vi "Add Block Diagram Content.vi"(8 "error in (no error)":errorcluster, 10 "Refs":T1, 11 "Module in":refnum<class "Module.lvclass">) -> (0 "error out":errorcluster, 2 "Local.Ref":refnum<vi>, 3 "Module out":refnum<class "Module.lvclass">)   [LabVIEW 2015, in "Module.lvclass"]
uses:
  Module.lvclass
  Loop/Block Diagram/BlockDiagram.Refs.ctl
  Loop/Block Diagram/Module.Refs.ctl
  <vilib>/Utility/miscctls.llb/LVPointTypeDef.ctl
  Loop/Block Diagram/Block Diagram.lvclass
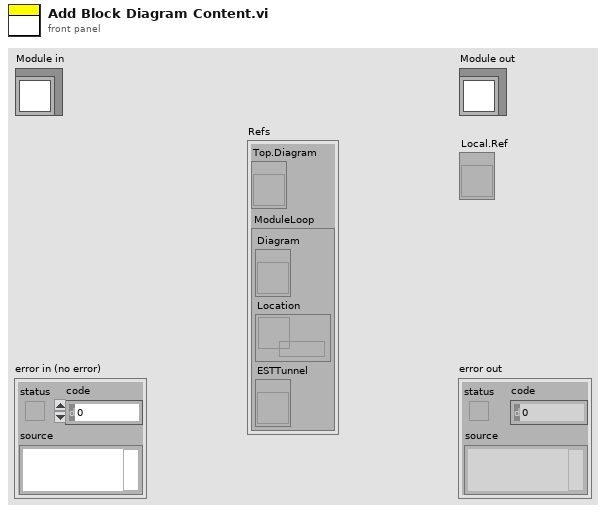
[diagram p1: front panel]
types:
  T1 = typedef "Block Diagram.lvclass/BlockDiagram.Refs.ctl" = cluster{"Top.Diagram":refnum<vi>, "ModuleLoop":T2}
  T2 = typedef "Block Diagram.lvclass/Module.Refs.ctl" = cluster{"Diagram":refnum<vi>, "Location":refnum<data-value>, "ESTTunnel":refnum<vi>}
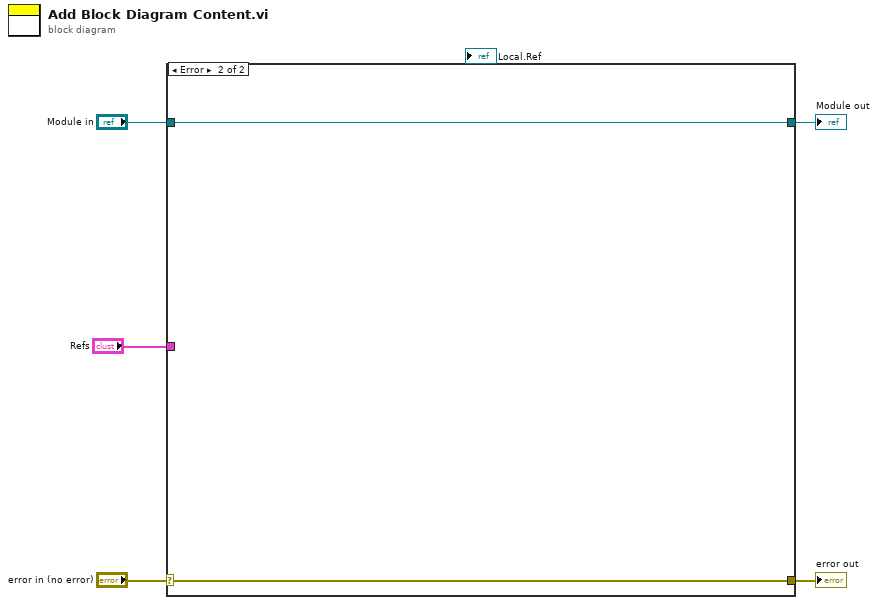
[diagram p0: block diagram]
diagram:
  n1 = case shown="Error" "error in (no error)" {
    selector: "error in (no error)" -> [w6 w9]
    tunnel: [w6 w9] -> w4
    tunnel: [w7 w8] -> w2
    tunnel: "Module in" -> [w7 w8]
    tunnel: "Refs" -> [_ _]
    frame No Error {
      # "Wire the error cluster across even in the \"No Error\"\ncase so that warnings get propagated."
    }
    frame Error {
    }
  }
  "error out" <- w4
  "Module out" <- w2
